vi "get_mode.vi"(8 "error in":errorcluster, 11 "VISA resource name":refnum<visa-resource-name>="COM1") -> (0 "error out":errorcluster, 3 "Response":string)   [LabVIEW 2020]
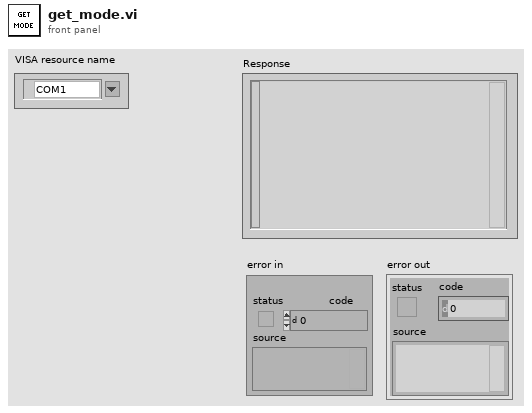
[diagram p1: front panel]
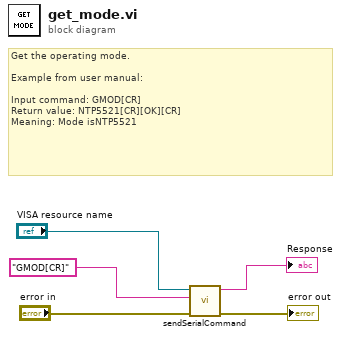
[diagram p0: block diagram]
diagram:
  # "Get the operating mode.\n\nExample from user manual:\n\nInput command: GMOD[CR]\nReturn value: NTP5521[CR][OK][CR]\nMeaning: Mode isNTP5521"
  n1 = call "sendSerialCommand.vi"("error in (no error)"="error in", "Command"="GMOD[CR]", "VISA resource name"="VISA resource name") -> ("error out"=→"error out":errorcluster, "Response"=→"Response":string)  [unwired: 7 in]
